vi "Replace Sweep Waveforms.vi"(10 "Channels New":T3[](array[typedef]) {"Table" format="%#_3p"; "Channel" min=1 max=16}, 11 "Sweep in":T4 {"sweepChannels"."Table" format="%#_1f"; "sweepChannels"."Channel" min=1 max=128; "sweepChannels"."Start" format="%#_6p"; "sweepChannels"."End" format="%#_6p"}) -> (3 "Sweep out":T4 {"sweepChannels"."Table" format="%#_1f"; "sweepChannels"."Channel" min=1 max=128; "sweepChannels"."Start" format="%#_6p"; "sweepChannels"."End" format="%#_6p"})   [LabVIEW 2019, in "Instrument.Lockin.lvlib" / "Instrument.Lockin.lvclass"]
uses:
  Instrument.Lockin.lvclass
  Instrument.DAQ/Typedefs/Sweep.Configuration--Cluster.ctl
  Instrument.DAQ/Typedefs/Sweep.Channel--Cluster--Array.ctl
  Instrument.DAQ/Typedefs/Sweep.Channel--Cluster.ctl
  Instrument.DAQ/Typedefs/Sweep.Pattern--Enum.ctl
  Typedefs/API/Lockin.setSweep_Table--cluster.ctl
  Instrument.DAQ/Instrument.DAQ.lvclass
panel:
  out "Array":T2(array[cluster])
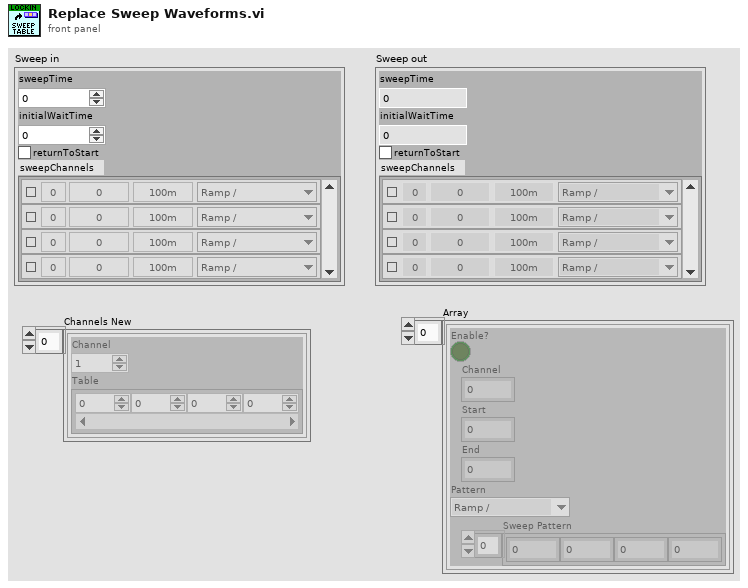
[diagram p1: front panel]
types:
  T1 = typedef "Instrument.Lockin.lvlib/Instrument.DAQ.lvclass/Sweep.Pattern--Enum.ctl" = enum16{"Ramp /", "Ramp /\\", "Smooth Ramp _/", "Smooth Ramp _/\\_", "Table"}
  T2 = cluster{"Enable?":bool, "Channel":u16, "Start":dbl, "End":dbl, "Pattern":T1, "Sweep Pattern":dbl[]}[]
  T3 = typedef "Instrument.Lockin.lvlib/Instrument.Lockin.lvclass/Lockin.setSweep_Table--cluster.ctl" = cluster{"Channel":i32, "Table":dbl[]}
  T4 = typedef "Instrument.Lockin.lvlib/Instrument.DAQ.lvclass/Sweep.Configuration--Cluster.ctl" = cluster{"sweepTime":dbl, "initialWaitTime":dbl, "returnToStart":bool, "sweepChannels":T5}
  T5 = typedef "Instrument.Lockin.lvlib/Instrument.DAQ.lvclass/Sweep.Channel--Cluster--Array.ctl" = T6[]
  T6 = typedef "Instrument.Lockin.lvlib/Instrument.DAQ.lvclass/Sweep.Channel--Cluster.ctl" = cluster{"Enable?":bool, "Channel":u16, "Start":dbl, "End":dbl, "Pattern":T1, "Table":dbl[]}
  T7 = cluster{"Enable?":bool, "Channel":u16, "Start":dbl, "End":dbl, "Pattern":T1, "Table":dbl[]}
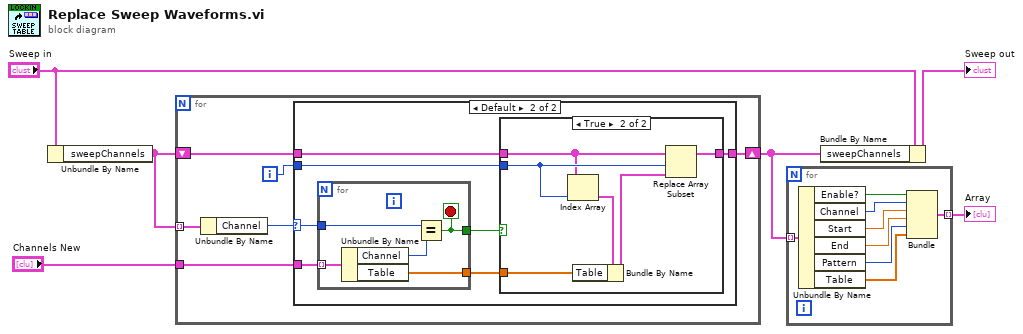
[diagram p0: block diagram]
diagram:
  n1 = Unbundle By Name("Sweep in") -> ("sweepChannels"=w4:T5)
  n2 = for {
    tunnel: "Channels New" -> [w9]
    shift-right: [w12] -> w2
    shift-left: w4 -> [w11]
    tunnel: w4 -> [w10] mode=indexing
    i -> [w7]
    n3 = Unbundle By Name(w10) -> ("Channel"=w8:u16)
    n4 = case shown="Default" w8 {
      selector: w8 -> [_ w17]
      tunnel: [w13 w20] -> w12
      tunnel: w11 -> [w13 w19]
      tunnel: w9 -> [_ w16]
      tunnel: w7 -> [_ w15]
      frame 0 {
      }
      frame Default {
        n5 = for {
          tunnel: w17 -> [w23]
          tunnel: [w25] -> w18
          tunnel: w16 -> [w24] mode=indexing
          tunnel: [w21] -> w14
          stop <- w25 stop-if-true
          n6 = Unbundle By Name(w24) -> ("Channel"=w22:i32, "Table"=w21:dbl[])
          n7 = Equal?(x=w23, y=w22) -> (x = y?=w25:bool)
        }
        n8 = case shown="True" w18 {
          tunnel: w19 -> [w26 w27]
          tunnel: [w26 w32] -> w20
          tunnel: w15 -> [_ w31]
          tunnel: w14 -> [_ w29]
          frame False {
          }
          frame True {
            n9 = Index Array(array=w27, index=w31) -> (element=w30:T6)
            n10 = Bundle By Name(cluster=w30, "Table"=w29) -> (w28:T6)
            n11 = Replace Array Subset(array=w27, new element=w28, index=w31) -> (w32:T5)
          }
        }
      }
    }
  }
  n12 = for {
    tunnel: w2 -> [w40] mode=indexing
    tunnel: [w33] -> w5 mode=indexing
    n13 = Unbundle By Name(w40) -> ("Enable?"=w39:bool, "Channel"=w38:u16, "Start"=w37:dbl, "End"=w36:dbl, "Pattern"=w35:T1, "Table"=w34:dbl[])
    n14 = Bundle("Enable?"=w39, "Channel"=w38, "Start"=w37, "End"=w36, "Pattern"=w35, "Table"=w34) -> (w33:T7)  [unwired: 1 in]
  }
  "Array" <- w5
  n15 = Bundle By Name(cluster="Sweep in", "sweepChannels"=w2) -> (→"Sweep out":T4)
